vi "Copy.vi"(8 "에러 입력":errorcluster caption="에러 입력(에러 없음)", 9 "소스 경로":path, 10 "타겟 경로":path) -> (0 "에러 출력":errorcluster, 3 "name":string)   [LabVIEW 2020]
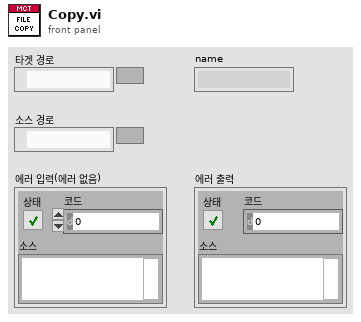
[diagram p1: front panel]
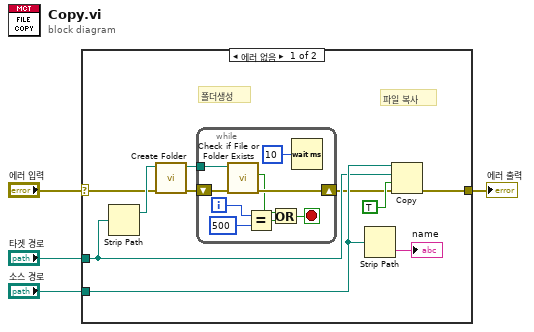
[diagram p0: block diagram]
diagram:
  n1 = case shown="에러 없음" "에러 입력" {
    selector: "에러 입력" -> [w5 w24]
    tunnel: [w14 w24] -> w4
    tunnel: "소스 경로" -> [w12 _]
    tunnel: "타겟 경로" -> [w10 _]
    frame No Error {
      # "파일 복사"
      # "폴더생성"
      n2 = Strip Path(path=w10) -> (stripped path=w8:path)  [unwired: 1 out]
      n3 = call "Create Folder.vi"("에러 입력"=w5, "폴더경로"=w8) -> ("error out"=w7:errorcluster, "dup path"=w6:path)  [unwired: 8 in]
      n4 = while {
        shift-right: [w22] -> w9
        shift-left: w7 -> [w23]
        tunnel: w6 -> [w21]
        i -> [w17]
        stop <- w19 stop-if-true
        n5 = call <vilib>:"Check if File or Folder Exists.vi"("error in (no error)"=w23, "path"=w21) -> ("error out"=w22:errorcluster, "file or folder exists?"=w20:bool)  [unwired: 7 in, 1 out]
        n6 = Equal?(x=w17, y=500) -> (x = y?=w18:bool)
        n7 = Or(x=w20, y=w18) -> (x .or. y?=w19:bool)
        n8 = Wait (ms)(milliseconds to wait=u32 10 ("대기 시간(ms)")) -> ()  [unwired: 1 out]
      }
      n9 = Strip Path(path=w12) -> (name=→"name":string)  [unwired: 1 out]
      n10 = Copy(8:w9, 9:TRUE ("덮어쓰기(거짓)"), 10:w10, 11:w12) -> (0:w14:errorcluster)  [unwired: 1 in, 2 out]
    }
    frame Error {
    }
  }
  "에러 출력" <- w4
